vi "Call_Lockin_and_IV.vi"(9 "Experiment folder name":string, 10 "Comments":string, 11 "Channels: AO in":T1) -> ()   [LabVIEW 2013]
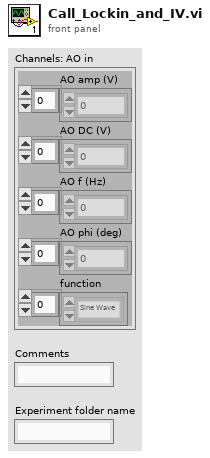
[diagram p1: front panel]
types:
  T1 = cluster{"AO amp (V)":dbl[], "AO DC (V)":dbl[], "AO f (Hz)":dbl[], "AO phi (deg)":dbl[], "function":enum16{"Sine Wave", "Triangle Wave", "Square Wave", "Sawtooth Wave"}[]}
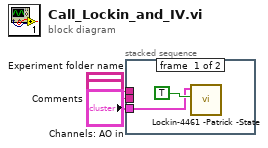
[diagram p0: block diagram]
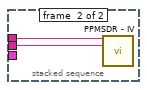
[diagram p2: hidden frame]
diagram:
  n1 = stacked-sequence {
    tunnel: "Experiment folder name" -> [_ w7]
    tunnel: "Comments" -> [_ w6]
    tunnel: "Channels: AO in" -> [w4 _]
    frame #0 {
      n2 = call <userlib>:"Lockin-4461 -Patrick -State.vi"("IV Curve Mode"=TRUE, "Channels: AO"=w4) -> ()  [unwired: 10 in]
    }
    frame #1 {
      n3 = call "PPMSDR - IV.vi"("Notes"=w6, "Experiment folder name"=w7) -> ()  [unwired: 10 in]
    }
  }
